vi "Freq Clamp And Note.vi"(3 "Frequency":dbl) -> (0 "Note":string, 1 "Clamped Freq":u32)   [LabVIEW 2011, in "LabVIEW Interface for Arduino.lvlib"]
uses:
  <vilib>/LabVIEW Interface for Arduino/LabVIEW Interface for Arduino.lvlib
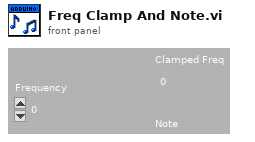
[diagram p1: front panel]
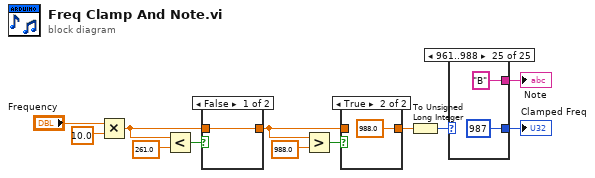
[diagram p0: block diagram]
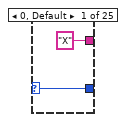
[diagram p2: hidden frame]
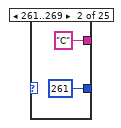
[diagram p3: hidden frame]
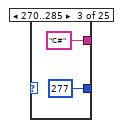
[diagram p4: hidden frame]
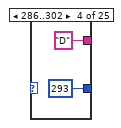
[diagram p5: hidden frame]
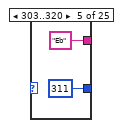
[diagram p6: hidden frame]
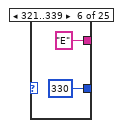
[diagram p7: hidden frame]
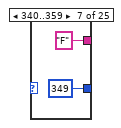
[diagram p8: hidden frame]
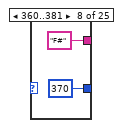
[diagram p9: hidden frame]
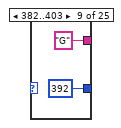
[diagram p10: hidden frame]
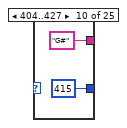
[diagram p11: hidden frame]
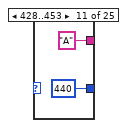
[diagram p12: hidden frame]
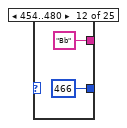
[diagram p13: hidden frame]
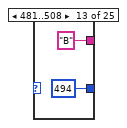
[diagram p14: hidden frame]
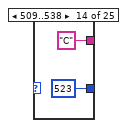
[diagram p15: hidden frame]
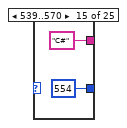
[diagram p16: hidden frame]
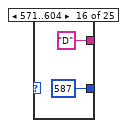
[diagram p17: hidden frame]
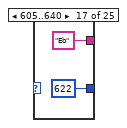
[diagram p18: hidden frame]
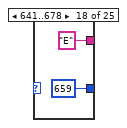
[diagram p19: hidden frame]
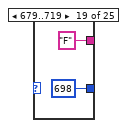
[diagram p20: hidden frame]
diagram:
  n1 = Multiply(x="Frequency", y=10.0) -> (x*y=w2:dbl)
  n2 = Less?(x=w2, y=261.0) -> (x < y?=w9:bool)
  n3 = case shown="False" w9 {
    tunnel: [w13 261.0 ("y")] -> w12
    tunnel: w2 -> [w13 _]
    frame False {
    }
    frame True {
    }
  }
  n4 = Greater?(x=w12, y=988.0) -> (0:w11:bool)
  n5 = case shown="True" w11 {
    tunnel: [w15 988.0 ("y")] -> w6
    tunnel: w12 -> [w15 _]
    frame False {
    }
    frame True {
    }
  }
  n6 = To Unsigned Long Integer(number=w6) -> (unsigned 32bit integer=w7:u32)
  n7 = case shown="961..988" w7 {
    selector: w7 -> [w18 _ _ _ _ _ _ _ _ _ _ _ _ _ _ _ _ _ _ _ _ _ _ _ _]
    tunnel: [w18 u32 261 u32 277 u32 293 u32 311 u32 330 u32 349 u32 370 u32 392 u32 415 u32 440 u32 466 u32 494 u32 523 u32 554 u32 587 u32 622 u32 659 u32 698 u32 740 u32 784 u32 830 u32 880 u32 932 u32 987] -> w5
    tunnel: ["X" "C" "C#" "D" "Eb" "E" "F" "F#" "G" "G#" "A" "Bb" "B" "C" "C#" "D" "Eb" "E" "F" "F#" "G" "G#" "A" "Bb" "B"] -> w4
    frame 0, Default {
    }
    frame 261..269 {
    }
    frame 270..285 {
    }
    frame 286..302 {
    }
    frame 303..320 {
    }
    frame 321..339 {
    }
    frame 340..359 {
    }
    frame 360..381 {
    }
    frame 382..403 {
    }
    frame 404..427 {
    }
    frame 428..453 {
    }
    frame 454..480 {
    }
    frame 481..508 {
    }
    frame 509..538 {
    }
    frame 539..570 {
    }
    frame 571..604 {
    }
    frame 605..640 {
    }
    frame 641..678 {
    }
    frame 679..719 {
    }
    frame 720..762 {
    }
    frame 763..807 {
    }
    frame 808..855 {
    }
    frame 856..906 {
    }
    frame 907..960 {
    }
    frame 961..988 {
    }
  }
  "Clamped Freq" <- w5
  "Note" <- w4
